vi "Timed Measurement.vi"() -> ()   [LabVIEW 2018]
uses:
  <vilib>/Instr/_visa.llb/VISA Configure Serial Port (Instr).vi
  <vilib>/Utility/file.llb/Write Delimited Spreadsheet (string).vi
  <vilib>/Utility/file.llb/Write Delimited Spreadsheet (I64).vi
panel:
  out "transposed array":i16[][](array[numeric])
  in  "Numarul persoanei":ext
  in  "Alegere Modul":u16(ring) items=["Stationare", "Mers normal", "Alergare", "Cadere", "Mers labartat"]
  out "Timer":dbl
  in  "Set Timer(Min)":dbl=2.0
  in  "Frecventa de esantionare [Hz]":dbl=50.0
  out "Calibration":T1
  out "read buffer":string
  in  "Clear Screen":bool
  in  "Bluetooth":refnum<visa-resource-name>="COM7"
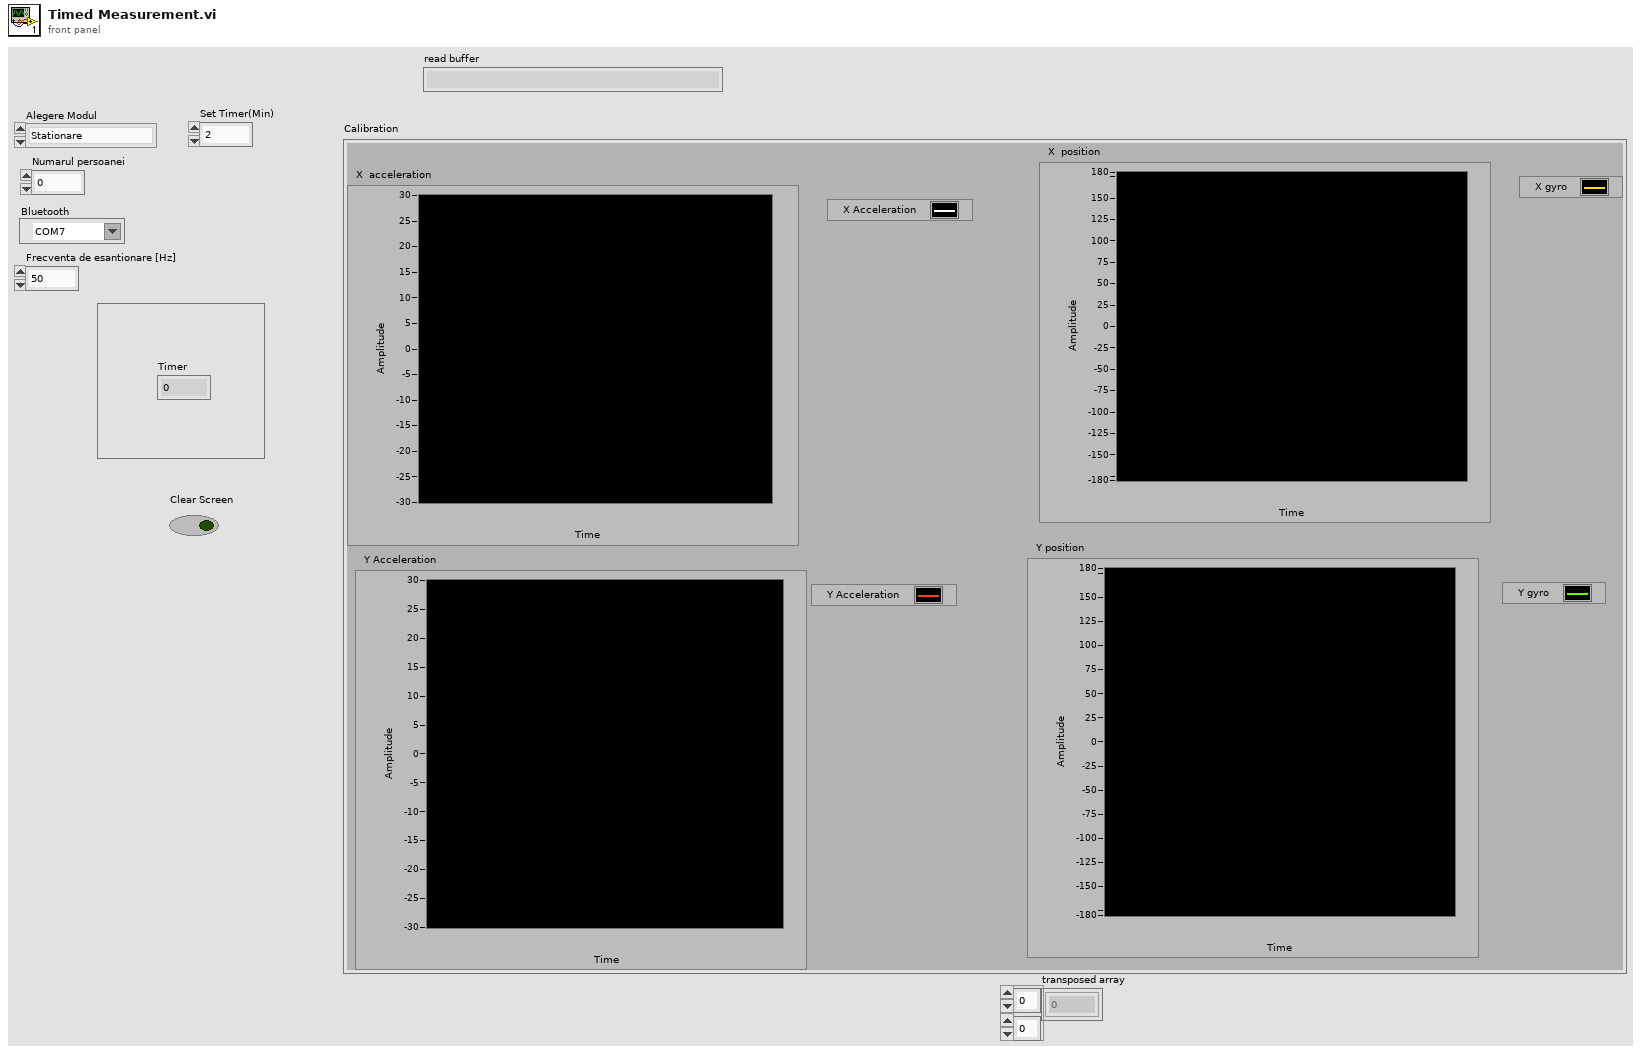
[diagram p1: front panel]
types:
  T1 = cluster{"X  acceleration":dbl, "Y Acceleration":dbl, "X  position":dbl, "Y position":dbl}
  T2 = typedef "imagedata.ctl" = cluster{"image type":i32, "image depth":i32, "image":u8[], "mask":u8[], "colors":u32[], "Rectangle":cluster{"left":i16, "top":i16, "right":i16, "bottom":i16}}
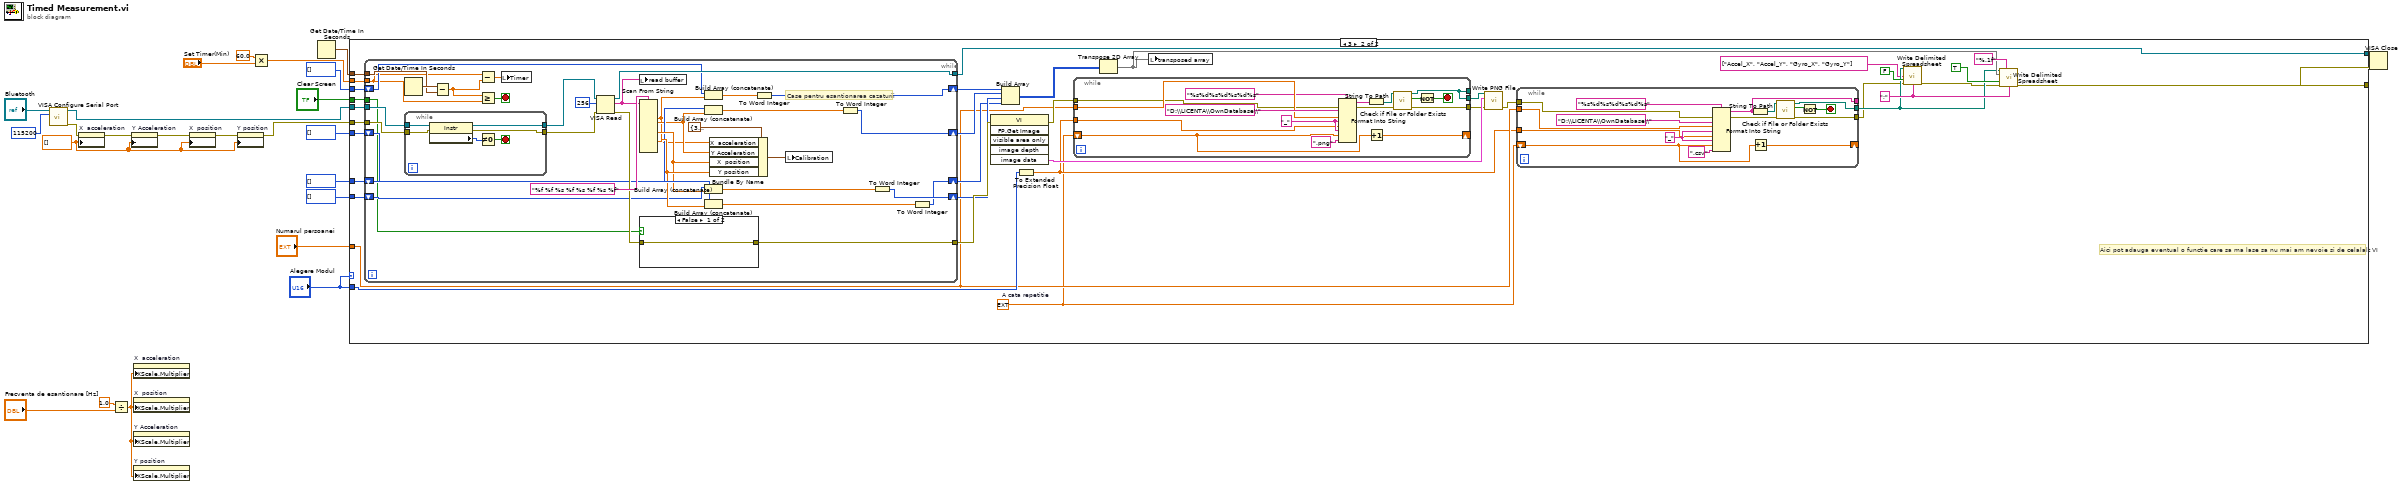
[diagram p0: block diagram]
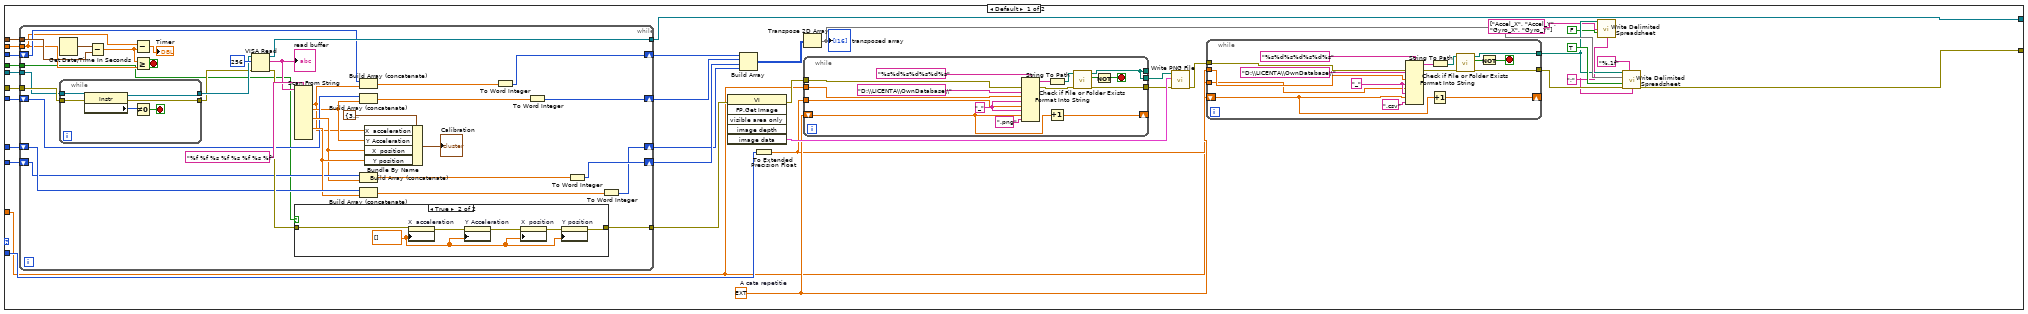
[diagram p2: hidden frame]
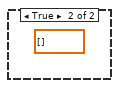
[diagram p4: hidden frame]
diagram:
  w17 = dbl[] [] ("History Data")
  n1 = call-poly "VISA Configure Serial Port"("VISA resource name"="Bluetooth", "baud rate (9600)"=u32 115200) -> ("VISA resource name out"=w23:refnum<visa-resource-name>, "error out"=w22:errorcluster)  [unwired: 12 in]
  n2 = property on="X  acceleration" class="WFChart (strict)"(error in=w22, "History Data"=w17) -> (error out=w21:errorcluster)  [unwired: 1 in, 1 out]
  n3 = Divide(x=1.0, y="Frecventa de esantionare [Hz]") -> (x/y=w16:dbl)
  n4 = property on="Y Acceleration" class="WFChart (strict)"(error in=w21, "History Data"=w17) -> (error out=w20:errorcluster)  [unwired: 1 in, 1 out]
  n5 = property on="X  acceleration" class="WFChart (strict)"("XScale.Multiplier"=w16) -> ()  [unwired: 2 in, 2 out]
  n6 = property on="X  position" class="WFChart (strict)"("XScale.Multiplier"=w16) -> ()  [unwired: 2 in, 2 out]
  n7 = property on="Y Acceleration" class="WFChart (strict)"("XScale.Multiplier"=w16) -> ()  [unwired: 2 in, 2 out]
  n8 = property on="Y position" class="WFChart (strict)"("XScale.Multiplier"=w16) -> ()  [unwired: 2 in, 2 out]
  n9 = property on="X  position" class="WFChart (strict)"(error in=w20, "History Data"=w17) -> (error out=w19:errorcluster)  [unwired: 1 in, 1 out]
  n10 = property on="Y position" class="WFChart (strict)"(error in=w19, "History Data"=w17) -> (error out=w18:errorcluster)  [unwired: 1 in, 1 out]
  n11 = Multiply(x=60.0, y="Set Timer(Min)") -> (x*y=w10:dbl)
  n12 = Get Date/Time In Seconds() -> (seconds since 1Jan1904=w13:timestamp)
  n13 = case shown="3" "Alegere Modul" {
    tunnel: w23 -> [w59 w174]
    tunnel: w18 -> [w58 w173]
    tunnel: w13 -> [w55 w170]
    tunnel: w10 -> [w54 w169]
    tunnel: "Alegere Modul" -> [w48 w164]
    tunnel: i16[] [] -> [w40 w158]
    tunnel: i16[] [] -> [w39 w157]
    tunnel: i16[] [] -> [w38 w156]
    tunnel: i16[] [] -> [w37 w155]
    tunnel: [w30 w140] -> w5
    tunnel: [w29 w150] -> w4
    tunnel: "Clear Screen" -> [w28 w149]
    tunnel: "Numarul persoanei" -> [w27 w144]
    frame Default {
      w41 = ext 1.0  # A cata repetitie
      w35 = ";" ("delimiter (\\t)")
      n14 = while {
        tunnel: w58 -> [w121]
        tunnel: w59 -> [w120]
        tunnel: [w116] -> w57
        tunnel: [w124] -> w29
        shift-right: [w93] -> w52
        shift-left: w37 -> [w115]
        tunnel: w55 -> [w111]
        tunnel: w54 -> [w101]
        shift-right: [w95] -> w53
        shift-left: w38 -> [w109]
        shift-right: [w96] -> w31
        shift-left: w39 -> [w105]
        shift-right: [w97] -> w32
        shift-left: w40 -> [w106]
        tunnel: w28 -> [w92]
        stop <- w110 stop-if-true
        n15 = Get Date/Time In Seconds() -> (seconds since 1Jan1904=w112:timestamp)
        n16 = while {
          tunnel: w121 -> [w139]
          tunnel: w120 -> [w138]
          tunnel: [w137] -> w119
          tunnel: [w136] -> w118
          stop <- w135 stop-if-true
          n17 = property class="Instr"(reference=w138, error in=w139) -> (reference out=w137:refnum<visa-resource-name>, error out=w136:errorcluster, "Serial Settings:Number of Bytes at Serial Port"=w134:u32)
          n18 = Not Equal To 0?(x=w134) -> (x != 0?=w135:bool)
        }
        n19 = Subtract(x=w112, y=w111) -> (x-y=w100:dbl)
        n20 = Subtract(x=w101, y=w100) -> (x-y=→"Timer":dbl)
        n21 = Greater Or Equal?(x=w100, y=w101) -> (x >= y?=w110:bool)
        n22 = VISA Read(VISA resource name=w119, byte count=u32 256, error in (no error)=w118) -> (VISA resource name out=w124:refnum<visa-resource-name>, read buffer=w122:string, error out=w117:errorcluster)  [unwired: 1 out]
        "read buffer" <- w122
        n23 = Scan From String(format string="%f %f %s %f %s %f %s %f", input string=w122) -> (output 1=w103:dbl, output 2=w104:dbl, output 4=w107:dbl, output 6=w114:dbl)  [unwired: 14 in, 3 out]
        n24 = case shown="True" w92 {
          tunnel: w117 -> [w127 w129]
          tunnel: [w127 w128] -> w116
          frame False {
          }
          frame True {
            w133 = dbl[] [] ("History Data")
            n25 = property on="X  acceleration" class="WFChart (strict)"(error in=w129, "History Data"=w133) -> (error out=w130:errorcluster)  [unwired: 1 in, 1 out]
            n26 = property on="Y Acceleration" class="WFChart (strict)"(error in=w130, "History Data"=w133) -> (error out=w131:errorcluster)  [unwired: 1 in, 1 out]
            n27 = property on="X  position" class="WFChart (strict)"(error in=w131, "History Data"=w133) -> (error out=w132:errorcluster)  [unwired: 1 in, 1 out]
            n28 = property on="Y position" class="WFChart (strict)"(error in=w132, "History Data"=w133) -> (error out=w128:errorcluster)  [unwired: 1 in, 1 out]
          }
        }
        n29 = Build Array (concatenate)(w105, w103) -> (w102:dbl[])
        n30 = Build Array (concatenate)(w106, w104) -> (w98:dbl[])
        n31 = Build Array (concatenate)(w109, w107) -> (w108:dbl[])
        n32 = Build Array (concatenate)(w115, w114) -> (w94:dbl[])
        n33 = Bundle By Name(cluster=T1 {"X  acceleration"=39.0, "Y Acceleration"=-79.0, "X  position"=180.0, "Y position"=92.0} ("Calibration"), "X  acceleration"=w103, "Y Acceleration"=w104, "X  position"=w107, "Y position"=w114) -> (→"Calibration":T1)
        n34 = To Word Integer(number=w102) -> (16bit integer=w96:i16[])
        n35 = To Word Integer(number=w98) -> (16bit integer=w97:i16[])
        n36 = To Word Integer(number=w108) -> (16bit integer=w95:i16[])
        n37 = To Word Integer(number=w94) -> (16bit integer=w93:i16[])
      }
      n38 = invoke class="VI" method="FP.Get Image"(error in=w57) -> (error out=w44:errorcluster, "image data"=w56:T2)  [unwired: 5 in, 4 out]
      n39 = Build Array(w31, w32, w53, w52) -> (w51:i16[][])
      n40 = To Extended Precision Float(1:w48) -> (0:w33:ext)
      n41 = Transpose 2D Array(2D array=w51) -> (transposed array=w50:i16[][])
      "transposed array" <- w50
      n42 = while {
        tunnel: w27 -> [w74]
        tunnel: w33 -> [w71]
        shift-right: [w64] -> _
        shift-left: w41 -> [w65]
        tunnel: [w63] -> w43
        tunnel: w44 -> [w62]
        tunnel: [w60] -> _
        tunnel: [w60] -> w42
        stop <- w67 stop-if-true
        w72 = "_"
        n43 = Format Into String(format string="%s%d%s%d%s%d%s", error in=w62, "D:\\LICENTA\\OwnDatabase\\", w74, w72, w71, w72, w65, ".png" ("input 7")) -> (resulting string=w70:string, error out=w66:errorcluster)  [unwired: 1 in]
        n44 = String To Path(string=w70) -> (path=w69:path)
        n45 = Increment(x=w65) -> (x+1=w64:ext)
        n46 = call <vilib>:"Check if File or Folder Exists.vi"("error in (no error)"=w66, "path"=w69) -> ("error out"=w63:errorcluster, "file or folder exists?"=w68:bool, "dup path"=w60:path)  [unwired: 7 in]
        n47 = Not(x=w68) -> (.not. x?=w67:bool)
      }
      n48 = call <vilib>:"Write PNG File.vi"("error in (no error)"=w43, "image data"=w56, "path to PNG file"=w42) -> ("error out"=w45:errorcluster)  [unwired: 7 in, 1 out]
      n49 = while {
        tunnel: w27 -> [w90]
        tunnel: w33 -> [w87]
        shift-right: [w80] -> _
        shift-left: w41 -> [w81]
        tunnel: [w79] -> w47
        tunnel: w45 -> [w78]
        tunnel: [w77] -> w36
        stop <- w83 stop-if-true
        w88 = "_"
        n50 = Format Into String(format string="%s%d%s%d%s%d%s", error in=w78, "D:\\LICENTA\\OwnDatabase\\", w90, w88, w87, w88, w81, ".csv" ("input 7")) -> (resulting string=w86:string, error out=w82:errorcluster)  [unwired: 1 in]
        n51 = String To Path(string=w86) -> (path=w85:path)
        n52 = Increment(x=w81) -> (x+1=w80:ext)
        n53 = call <vilib>:"Check if File or Folder Exists.vi"("error in (no error)"=w82, "path"=w85) -> ("error out"=w79:errorcluster, "file or folder exists?"=w84:bool, "dup path"=w77:path)  [unwired: 7 in]
        n54 = Not(x=w84) -> (.not. x?=w83:bool)
      }
      n55 = call-poly <vilib>:"Write Delimited Spreadsheet.vi"("file path (dialog if empty)"=w36, "1D data"=string[] ["Accel_X", "Accel_Y", "Gyro_X", "Gyro_Y"] ("Array"), "append to file? (new file:F)"=FALSE, "delimiter (\\t)"=w35) -> ()  [unwired: 10 in, 2 out]
      n56 = call-poly <vilib>:"Write Delimited Spreadsheet.vi"("file path (dialog if empty)"=w36, "format (%d)"="%.1f" ("format (%.3f)"), "2D data"=w50, "append to file? (new file:F)"=TRUE, "error in (no error)"=w47, "delimiter (\\t)"=w35) -> ("error out"=w30:errorcluster)  [unwired: 8 in, 1 out]
    }
    frame 3 {
      w142 = ext 1.0  # A cata repetitie
      w154 = ";" ("delimiter (\\t)")
      # "Aici pot adauga eventual o functie care sa ma lase sa nu mai am nevoie si de celalalt VI"
      n57 = while {
        tunnel: w173 -> [w237]
        tunnel: w174 -> [w236]
        tunnel: [w232] -> w172
        tunnel: [w239] -> w150
        shift-right: [w213] -> w167
        shift-left: w155 -> [w231]
        tunnel: w170 -> [w228]
        tunnel: w169 -> [w219]
        shift-right: [w215] -> w168
        shift-left: w156 -> [w226]
        shift-right: [w209] -> w151
        shift-left: w157 -> [w222]
        shift-right: [w216] -> w152
        shift-left: w158 -> [w223]
        tunnel: w149 -> [w210]
        stop <- w227 stop-if-true
        # "Case pentru esantionarea cazaturii"
        n58 = Get Date/Time In Seconds() -> (seconds since 1Jan1904=w229:timestamp)
        n59 = while {
          tunnel: w237 -> [w248]
          tunnel: w236 -> [w247]
          tunnel: [w246] -> w235
          tunnel: [w245] -> w234
          stop <- w244 stop-if-true
          n60 = property class="Instr"(reference=w247, error in=w248) -> (reference out=w246:refnum<visa-resource-name>, error out=w245:errorcluster, "Serial Settings:Number of Bytes at Serial Port"=w243:u32)
          n61 = Not Equal To 0?(x=w243) -> (x != 0?=w244:bool)
        }
        n62 = Subtract(x=w229, y=w228) -> (x-y=w218:dbl)
        n63 = Subtract(x=w219, y=w218) -> (x-y=w211:dbl)
        n64 = Greater Or Equal?(x=w218, y=w219) -> (x >= y?=w227:bool)
        n65 = local write "Timer"(w211) -> ()
        n66 = VISA Read(VISA resource name=w235, byte count=u32 256, error in (no error)=w234) -> (VISA resource name out=w239:refnum<visa-resource-name>, read buffer=w207:string, error out=w233:errorcluster)  [unwired: 1 out]
        n67 = local write "read buffer"(w207) -> ()
        n68 = Scan From String(format string="%f %f %s %f %s %f %s %f", input string=w207) -> (output 1=w208:dbl, output 2=w221:dbl, output 4=w224:dbl, output 6=w230:dbl)  [unwired: 14 in, 3 out]
        n69 = case shown="False" w210 {
          tunnel: w233 -> [w242 _]
          tunnel: [w242 _] -> w232
          frame False {
          }
          frame True {
            (unwired) dbl[] [] ("History Data")
          }
        }
        n70 = Build Array (concatenate)(w222, w208) -> (w220:dbl[])
        n71 = Build Array (concatenate)(w223, w221) -> (w217:dbl[])
        n72 = Build Array (concatenate)(w226, w224) -> (w225:dbl[])
        n73 = Build Array (concatenate)(w231, w230) -> (w214:dbl[])
        n74 = Bundle By Name(cluster=T1 {"X  acceleration"=39.0, "Y Acceleration"=-79.0, "X  position"=180.0, "Y position"=92.0} ("Calibration"), "X  acceleration"=w208, "Y Acceleration"=w221, "X  position"=w224, "Y position"=w230) -> (w212:T1)
        n75 = To Word Integer(number=w220) -> (16bit integer=w209:i16[])
        n76 = local write "Calibration"(w212) -> ()
        n77 = To Word Integer(number=w217) -> (16bit integer=w216:i16[])
        n78 = To Word Integer(number=w225) -> (16bit integer=w215:i16[])
        n79 = To Word Integer(number=w214) -> (16bit integer=w213:i16[])
      }
      n80 = invoke class="VI" method="FP.Get Image"(error in=w172) -> (error out=w161:errorcluster, "image data"=w171:T2)  [unwired: 5 in, 4 out]
      n81 = Build Array(w151, w152, w168, w167) -> (w166:i16[][])
      n82 = To Extended Precision Float(1:w164) -> (0:w143:ext)
      n83 = while {
        tunnel: w144 -> [w189]
        tunnel: w143 -> [w186]
        shift-right: [w179] -> _
        shift-left: w142 -> [w180]
        tunnel: [w178] -> w160
        tunnel: w161 -> [w177]
        tunnel: [w175] -> _
        tunnel: [w175] -> w159
        stop <- w182 stop-if-true
        w187 = "_"
        n84 = Format Into String(format string="%s%d%s%d%s%d%s", error in=w177, "D:\\LICENTA\\OwnDatabase\\", w189, w187, w186, w187, w180, ".png" ("input 7")) -> (resulting string=w185:string, error out=w181:errorcluster)  [unwired: 1 in]
        n85 = String To Path(string=w185) -> (path=w184:path)
        n86 = Increment(x=w180) -> (x+1=w179:ext)
        n87 = call <vilib>:"Check if File or Folder Exists.vi"("error in (no error)"=w181, "path"=w184) -> ("error out"=w178:errorcluster, "file or folder exists?"=w183:bool, "dup path"=w175:path)  [unwired: 7 in]
        n88 = Not(x=w183) -> (.not. x?=w182:bool)
      }
      n89 = Transpose 2D Array(2D array=w166) -> (transposed array=w148:i16[][])
      n90 = local write "transposed array"(w148) -> ()
      n91 = call <vilib>:"Write PNG File.vi"("error in (no error)"=w160, "image data"=w171, "path to PNG file"=w159) -> ("error out"=w162:errorcluster)  [unwired: 7 in, 1 out]
      n92 = while {
        tunnel: w144 -> [w205]
        tunnel: w143 -> [w202]
        shift-right: [w196] -> _
        shift-left: w142 -> [w197]
        tunnel: [w195] -> w145
        tunnel: w162 -> [w194]
        tunnel: [w193] -> w147
        tunnel: [w191] -> _
        stop <- w199 stop-if-true
        w203 = "_"
        n93 = Format Into String(format string="%s%d%s%d%s%d%s", error in=w194, "D:\\LICENTA\\OwnDatabase\\", w205, w203, w202, w203, w197, ".csv" ("input 7")) -> (resulting string=w191:string, error out=w198:errorcluster)  [unwired: 1 in]
        n94 = String To Path(string=w191) -> (path=w201:path)
        n95 = Increment(x=w197) -> (x+1=w196:ext)
        n96 = call <vilib>:"Check if File or Folder Exists.vi"("error in (no error)"=w198, "path"=w201) -> ("error out"=w195:errorcluster, "file or folder exists?"=w200:bool, "dup path"=w193:path)  [unwired: 7 in]
        n97 = Not(x=w200) -> (.not. x?=w199:bool)
      }
      n98 = call-poly <vilib>:"Write Delimited Spreadsheet.vi"("file path (dialog if empty)"=w147, "1D data"=string[] ["Accel_X", "Accel_Y", "Gyro_X", "Gyro_Y"] ("Array"), "append to file? (new file:F)"=FALSE, "error in (no error)"=w145, "delimiter (\\t)"=w154) -> ("error out"=w146:errorcluster)  [unwired: 9 in, 1 out]
      n99 = call-poly <vilib>:"Write Delimited Spreadsheet.vi"("file path (dialog if empty)"=w147, "format (%d)"="%.1f" ("format (%.3f)"), "2D data"=w148, "append to file? (new file:F)"=TRUE, "error in (no error)"=w146, "delimiter (\\t)"=w154) -> ("error out"=w140:errorcluster)  [unwired: 8 in, 1 out]
    }
  }
  n100 = VISA Close(VISA resource name=w4, error in (no error)=w5) -> ()  [unwired: 1 out]
